vi "字符转换C代码.vi"(11 "扫码枪字符识别":string="C0C01B2473002") -> (3 "子字符串 4":string)   [LabVIEW 2017]
panel:
  out "子字符串 3":string
  out "子字符串 2":string
  out "子字符串":string
  # "C.08.002"
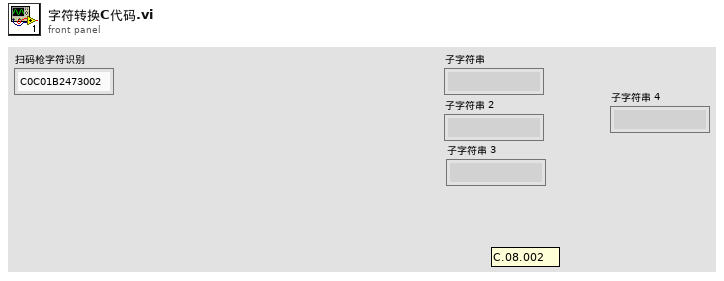
[diagram p1: front panel]
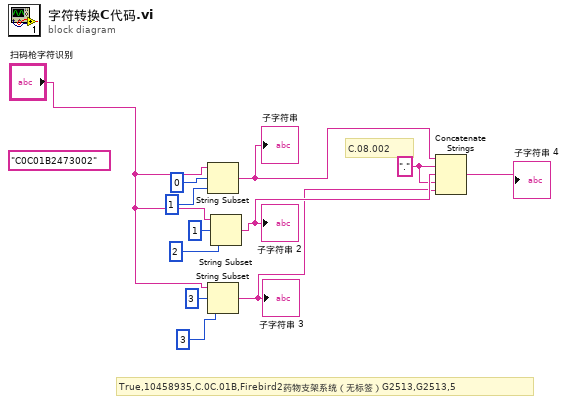
[diagram p0: block diagram]
diagram:
  w4 = "." ("字符串")
  (unwired) "C0C01B2473002" ("扫码枪字符识别")
  # "True,10458935,C.0C.01B,Firebird2药物支架系统（无标签）G2513,G2513,5"
  # "C.08.002"
  n1 = String Subset(string="扫码枪字符识别", offset (0)=0 ("偏移量(0)"), length (rest)=1 ("长度（剩余）")) -> (substring=w6:string)
  "子字符串" <- w6
  n2 = String Subset(string="扫码枪字符识别", offset (0)=3 ("偏移量(0)"), length (rest)=3 ("长度（剩余）")) -> (substring=w3:string)
  "子字符串 3" <- w3
  n3 = String Subset(string="扫码枪字符识别", offset (0)=1 ("偏移量(0)"), length (rest)=2 ("长度（剩余）")) -> (substring=w5:string)
  "子字符串 2" <- w5
  n4 = Concatenate Strings(w6, w4, w5, w4, w3) -> (→"子字符串 4":string)
